vi "Find Max Min Value.vi"(8 "error in (no error)":errorcluster, 10 "ImageIn":T1, 11 "ImageHandler in":refnum<class "ImageHandler.lvclass">) -> (0 "error out":errorcluster, 1 "Maximal Value":i32, 2 "Minimal Value":i32, 3 "ImageHandler out":refnum<class "ImageHandler.lvclass">)   [LabVIEW 2022 SP3, in "ImageHandler.lvlib" / "ImageHandler.lvclass"]
uses:
  ImageHandler.lvclass
  <vilib>/vision/Image Controls.llb/IMAQ Image.ctl
  ImageHandler.lvclass/ImageHandler.ctl
  <vilib>/vision/NI_Vision_Development_Module.lvlib
  <resource>/objmgr/IMAQImage.rc
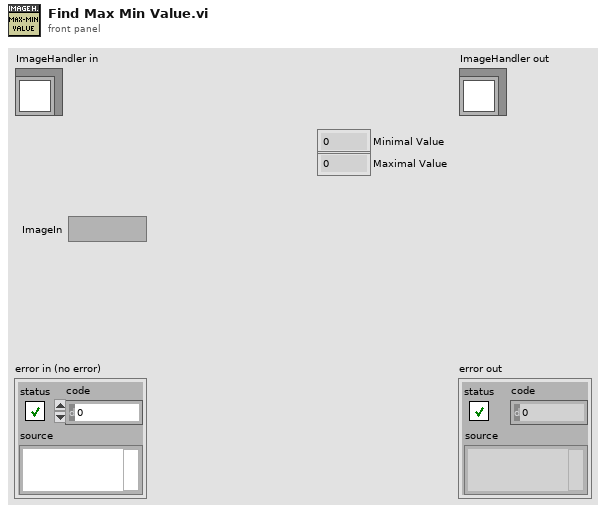
[diagram p1: front panel]
types:
  T1 = typedef "IMAQ Image.ctl" = refnum<image>
  T2 = cluster{"histogram":u32[], "Minimal Value":sgl, "Maximal Value":sgl, "Starting Value":sgl, "Interval Width":sgl, "Mean Value":sgl, "Standard  Variation":sgl, "Area (pixels)":i32}
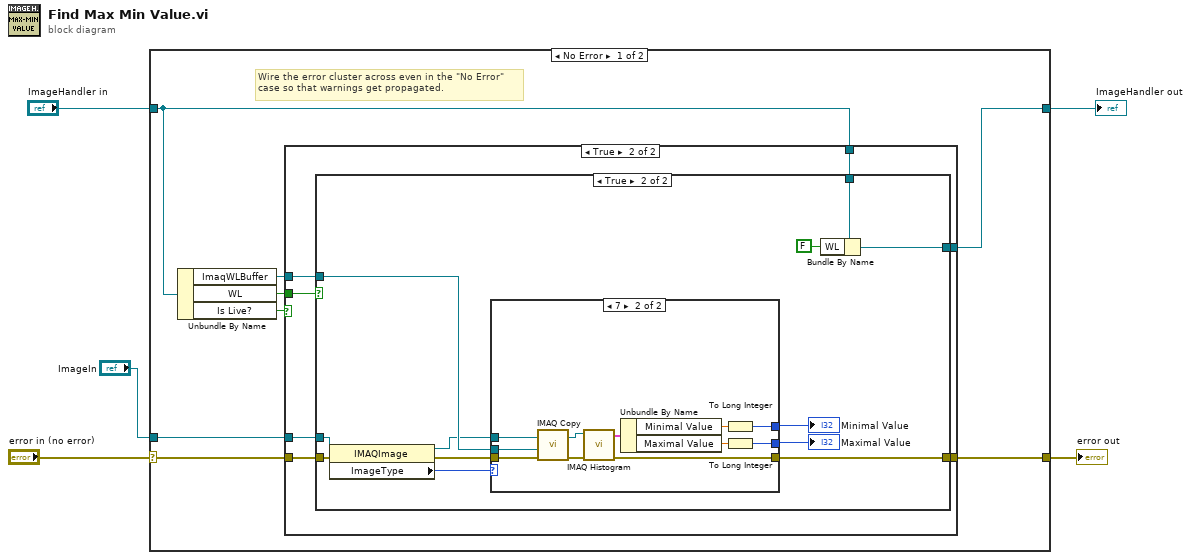
[diagram p0: block diagram]
diagram:
  n1 = case shown="No Error" "error in (no error)" {
    selector: "error in (no error)" -> [w13 w50]
    tunnel: [w12 w50] -> w4
    tunnel: [w6 w49] -> w2
    tunnel: "ImageHandler in" -> [w7 w49]
    tunnel: "ImageIn" -> [w8 _]
    frame No Error {
      # "Wire the error cluster across even in the \"No Error\"\ncase so that warnings get propagated."
      n2 = Unbundle By Name(w7) -> ("ImaqWLBuffer"=w9:T1, "WL"=w10:bool, "Is Live?"=w11:bool)
      n3 = case shown="True" w11 {
        tunnel: w13 -> [w15 w21]
        tunnel: [w15 w20] -> w12
        tunnel: w10 -> [_ w22]
        tunnel: w9 -> [_ w19]
        tunnel: w8 -> [_ w18]
        tunnel: w7 -> [w14 w17]
        tunnel: [w14 w16] -> w6
        frame False {
        }
        frame True {
          n4 = case shown="True" w22 {
            tunnel: w21 -> [w24 w36]
            tunnel: [w24 w34] -> w20
            tunnel: w19 -> [_ w35]
            tunnel: w18 -> [_ w29]
            tunnel: w17 -> [w23 w33]
            tunnel: [w23 w32] -> w16
            frame False {
            }
            frame True {
              n5 = property class="IMAQImage"(reference=w29, error in=w36) -> (reference out=w28:T1, error out=w30:errorcluster, "ImageType"=w27:u32)
              n6 = case shown="7" w27 {
                tunnel: w35 -> [_ w47]
                tunnel: [w37 w46] -> w34
                tunnel: w30 -> [w37 w41]
                tunnel: w28 -> [_ w40]
                tunnel: [_ w39] -> w26
                tunnel: [_ w38] -> w25
                frame 0, Default {
                }
                frame 7 {
                  n7 = call "IMAQ Copy"("error in (no error)"=w41, "Image Dst"=w47, "Image Src"=w40) -> ("error out"=w48:errorcluster, "Image Dst Out"=w45:T1)  [unwired: 3 in]
                  n8 = call "IMAQ Histogram"("error in (no error)"=w48, "Image"=w45) -> ("error out"=w46:errorcluster, "Histogram Report"=w44:T2)  [unwired: 8 in]
                  n9 = Unbundle By Name(w44) -> ("Minimal Value"=w43:sgl, "Maximal Value"=w42:sgl)
                  n10 = To Long Integer(number=w43) -> (32bit integer=w38:i32)
                  n11 = To Long Integer(number=w42) -> (32bit integer=w39:i32)
                }
              }
              "Minimal Value" <- w25
              "Maximal Value" <- w26
              n12 = Bundle By Name(cluster=w33, "WL"=FALSE) -> (w32:refnum<class "ImageHandler.lvclass">)
            }
          }
        }
      }
    }
    frame Error {
    }
  }
  "error out" <- w4
  "ImageHandler out" <- w2
